vi "Example DHTxx Reading.vi"() -> ()   [LabVIEW 2014]
uses:
  vi.lib/Q-WaveSystems/QwaveSys Raspberry Pi for LabVIEW Home-Education/QwaveSys Raspberry Pi Library.lvlib
panel:
  out "Active":bool
  out "f":dbl
  out "c":dbl
  out "h":dbl
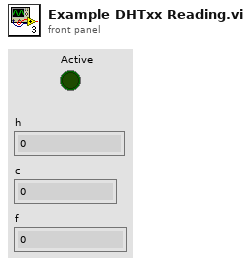
[diagram p1: front panel]
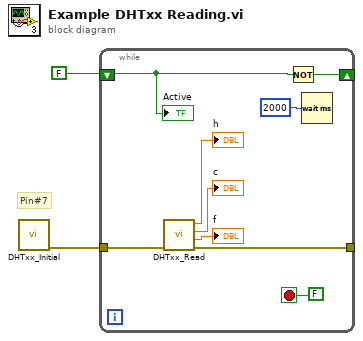
[diagram p0: block diagram]
diagram:
  # "Pin#7"
  n1 = call "DHTxx_Initial.vi"() -> ("error out"=w2:errorcluster)  [unwired: 10 in, 1 out]
  n2 = while {
    tunnel: w2 -> [w9]
    tunnel: [w8] -> _
    shift-right: [w4] -> _
    shift-left: FALSE -> [w3]
    stop <- FALSE stop-if-true
    n3 = call "DHTxx_Read.vi"("error in (no error)"=w9) -> ("error out"=w8:errorcluster, "f"=→"f":sgl, "c"=→"c":sgl, "h"=→"h":sgl)  [unwired: 7 in]
    n4 = Not(x=w3) -> (.not. x?=w4:bool)
    n5 = Wait (ms)(milliseconds to wait=u32 2000) -> ()  [unwired: 1 out]
    "Active" <- w3
  }
